vi "Address Query.vi"(8 "Error In (No Error)":errorcluster, 11 "RS232 Port In":refnum<visa-resource-name>) -> (0 "Error Out":errorcluster, 1 "Sensor Response?":bool, 2 "Sensor Address Out":string, 3 "RS232 Port Out":refnum<visa-resource-name>)   [LabVIEW 2016, in "SDI-12.lvlib"]
doc: "Sends an SDI-12 Query Address broadcast to all sensors on the SDI-12 line. However, this VI has only been designed to handle a single sensor response. An orderly multi-sensor reply is beyond the scope of the SDI-12 protocol."
uses:
  SDI-12.lvlib
panel:
  # "WARNING: \nIt is highly recommended that only one sensor is connected to your SDI-12 cable.  Otherwise, \nthis command will cause network congestion.  If your sensors are all able to reply in an orderly fashion, \nyou will need to edit this VI to handle multiple responses."
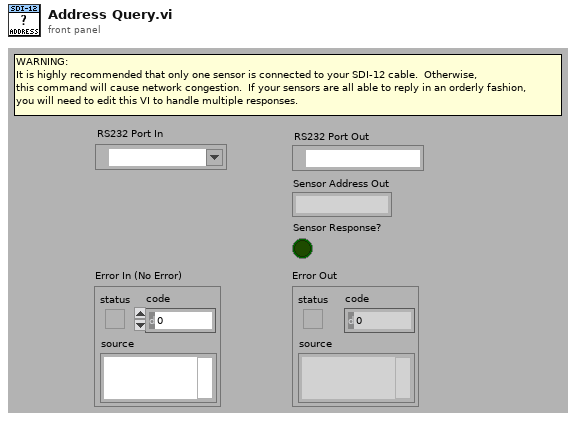
[diagram p1: front panel]
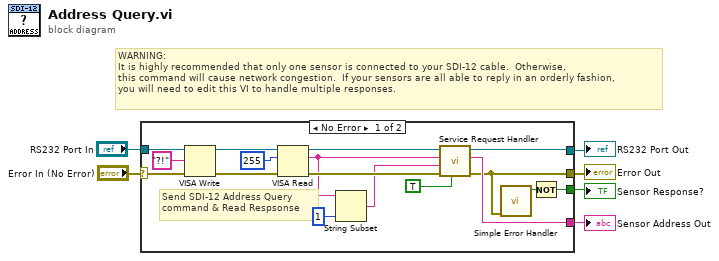
[diagram p0: block diagram]
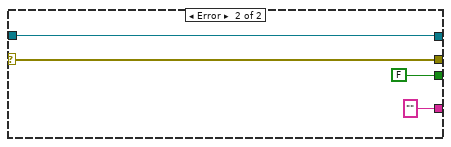
[diagram p2: hidden frame]
diagram:
  # "WARNING: \nIt is highly recommended that only one sensor is connected to your SDI-12 cable.  Otherwise, \nthis command will cause network congestion.  If your sensors are all able to reply in an orderly fashion, \nyou will need to edit this VI to handle multiple responses."
  n1 = case shown="No Error" "Error In (No Error)" {
    selector: "Error In (No Error)" -> [w18 w26]
    tunnel: [w8 FALSE ("sensor response?")] -> w5
    tunnel: [w7 w26] -> w1
    tunnel: "RS232 Port In" -> [w15 w25]
    tunnel: [w14 w25] -> w3
    tunnel: [w13 "" ("sensor address out")] -> w2
    frame No Error {
      # "Send SDI-12 Address Query \ncommand & Read Respsonse"
      n2 = VISA Write(VISA resource name=w15, write buffer="?!", error in (no error)=w18) -> (VISA resource name out=w23:refnum<visa-resource-name>, error out=w22:errorcluster)  [unwired: 1 out]
      n3 = VISA Read(VISA resource name=w23, byte count=u32 255, error in (no error)=w22) -> (VISA resource name out=w17:refnum<visa-resource-name>, read buffer=w12:string, error out=w20:errorcluster)  [unwired: 1 out]
      n4 = String Subset(string=w12, length (rest)=1 ("length (rest)")) -> (substring=w10:string)  [unwired: 1 in]
      n5 = call "Service Request Handler.vi"("Check address? (False)"=TRUE ("Check address? (false)"), "Error In (No Error)"=w20, "Expected Sensor Address (a)"=w10, "Service Request"=w12, "RS232 Port In"=w17) -> ("Error Out"=w7:errorcluster, "Sensor Address Out"=w13:string, "RS232 Port Out"=w14:refnum<visa-resource-name>)  [unwired: 3 in, 1 out]
      n6 = call <vilib>:"Simple Error Handler.vi"("error in (no error)"=w7) -> ("error?"=w9:bool)  [unwired: 4 in, 4 out]
      n7 = Not(x=w9) -> (.not. x?=w8:bool)
    }
    frame Error {
    }
  }
  "Sensor Response?" <- w5
  "RS232 Port Out" <- w3
  "Sensor Address Out" <- w2
  "Error Out" <- w1
